vi "Interpret Driver Controls.vi"() -> ()   [LabVIEW 2018]
uses:
  <vilib>/Rock Robotics/WPI/DriverStation/WPI_DriverStationDerivedRobotMode.ctl
  Robot Global Data.vi
  SubSystems/Controllers/Driver Controller/Driver Controller Global.vi
  SubSystems/Drive Train/Drive Train Global.vi
  SubSystems/Lift/Lift Global.vi
  SubSystems/Controllers/Manipulator Controlller/Manipulator Controller Global.vi
  SubSystems/HAB Climber/HAB Climber Global.vi
  <vilib>/addons/control/pid/pid.llb/PID (DBL).vi
  SubSystems/Cargo Intake/Cargo Intake Global.vi
  SubSystems/Hatch Panel Intake/Hatch Panel Intake Global.vi
  <vilib>/addons/control/pid/NI_PID_pid.lvlib
panel:
  in  "Last Move Deadband":u32=500
  in  "Last Time Auto":u32=1171826
  in  "Camera Tracking":T1={"proportional gain (Kc)"=0.06, "integral time (Ti, min)"=0.0, "derivative time (Td, min)"=0.0}
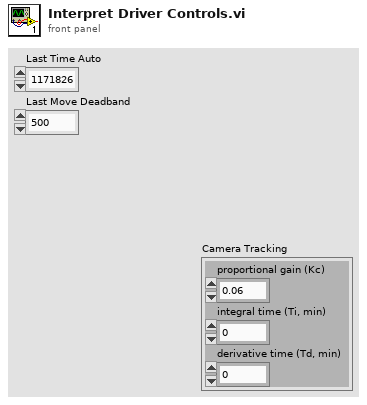
[diagram p1: front panel]
types:
  T1 = cluster{"proportional gain (Kc)":dbl, "integral time (Ti, min)":dbl, "derivative time (Td, min)":dbl}
  T2 = enum16{"Manual", "Hatch Panel Zone 1", "Hatch Panel Zone 2", "Hatch Panel Zone 3", "Cargo Zone 1", "Cargo Zone 2", "Cargo Zone 3", "Cargo Ship Zone"}
  T3 = enum16{"Hatch Panel Zone 1", "Hatch Panel Zone 2", "Hatch Panel Zone 3", "Cargo Zone 1", "Cargo Zone 2", "Cargo Zone 3", "Cargo Ship Zone"}
  T4 = cluster{"Rollover":dbl, "Yaw":dbl, "Cont Yaw":dbl}
  T5 = typedef "WPI_DriverStationDerivedRobotMode.ctl" = enum16{"Init", "Execute", "Stop"}
  T6 = cluster{"offsetAngle H":dbl, "offsetAngle V":dbl, "area":dbl, "skew":dbl, "validTarget":dbl, "latency":dbl}
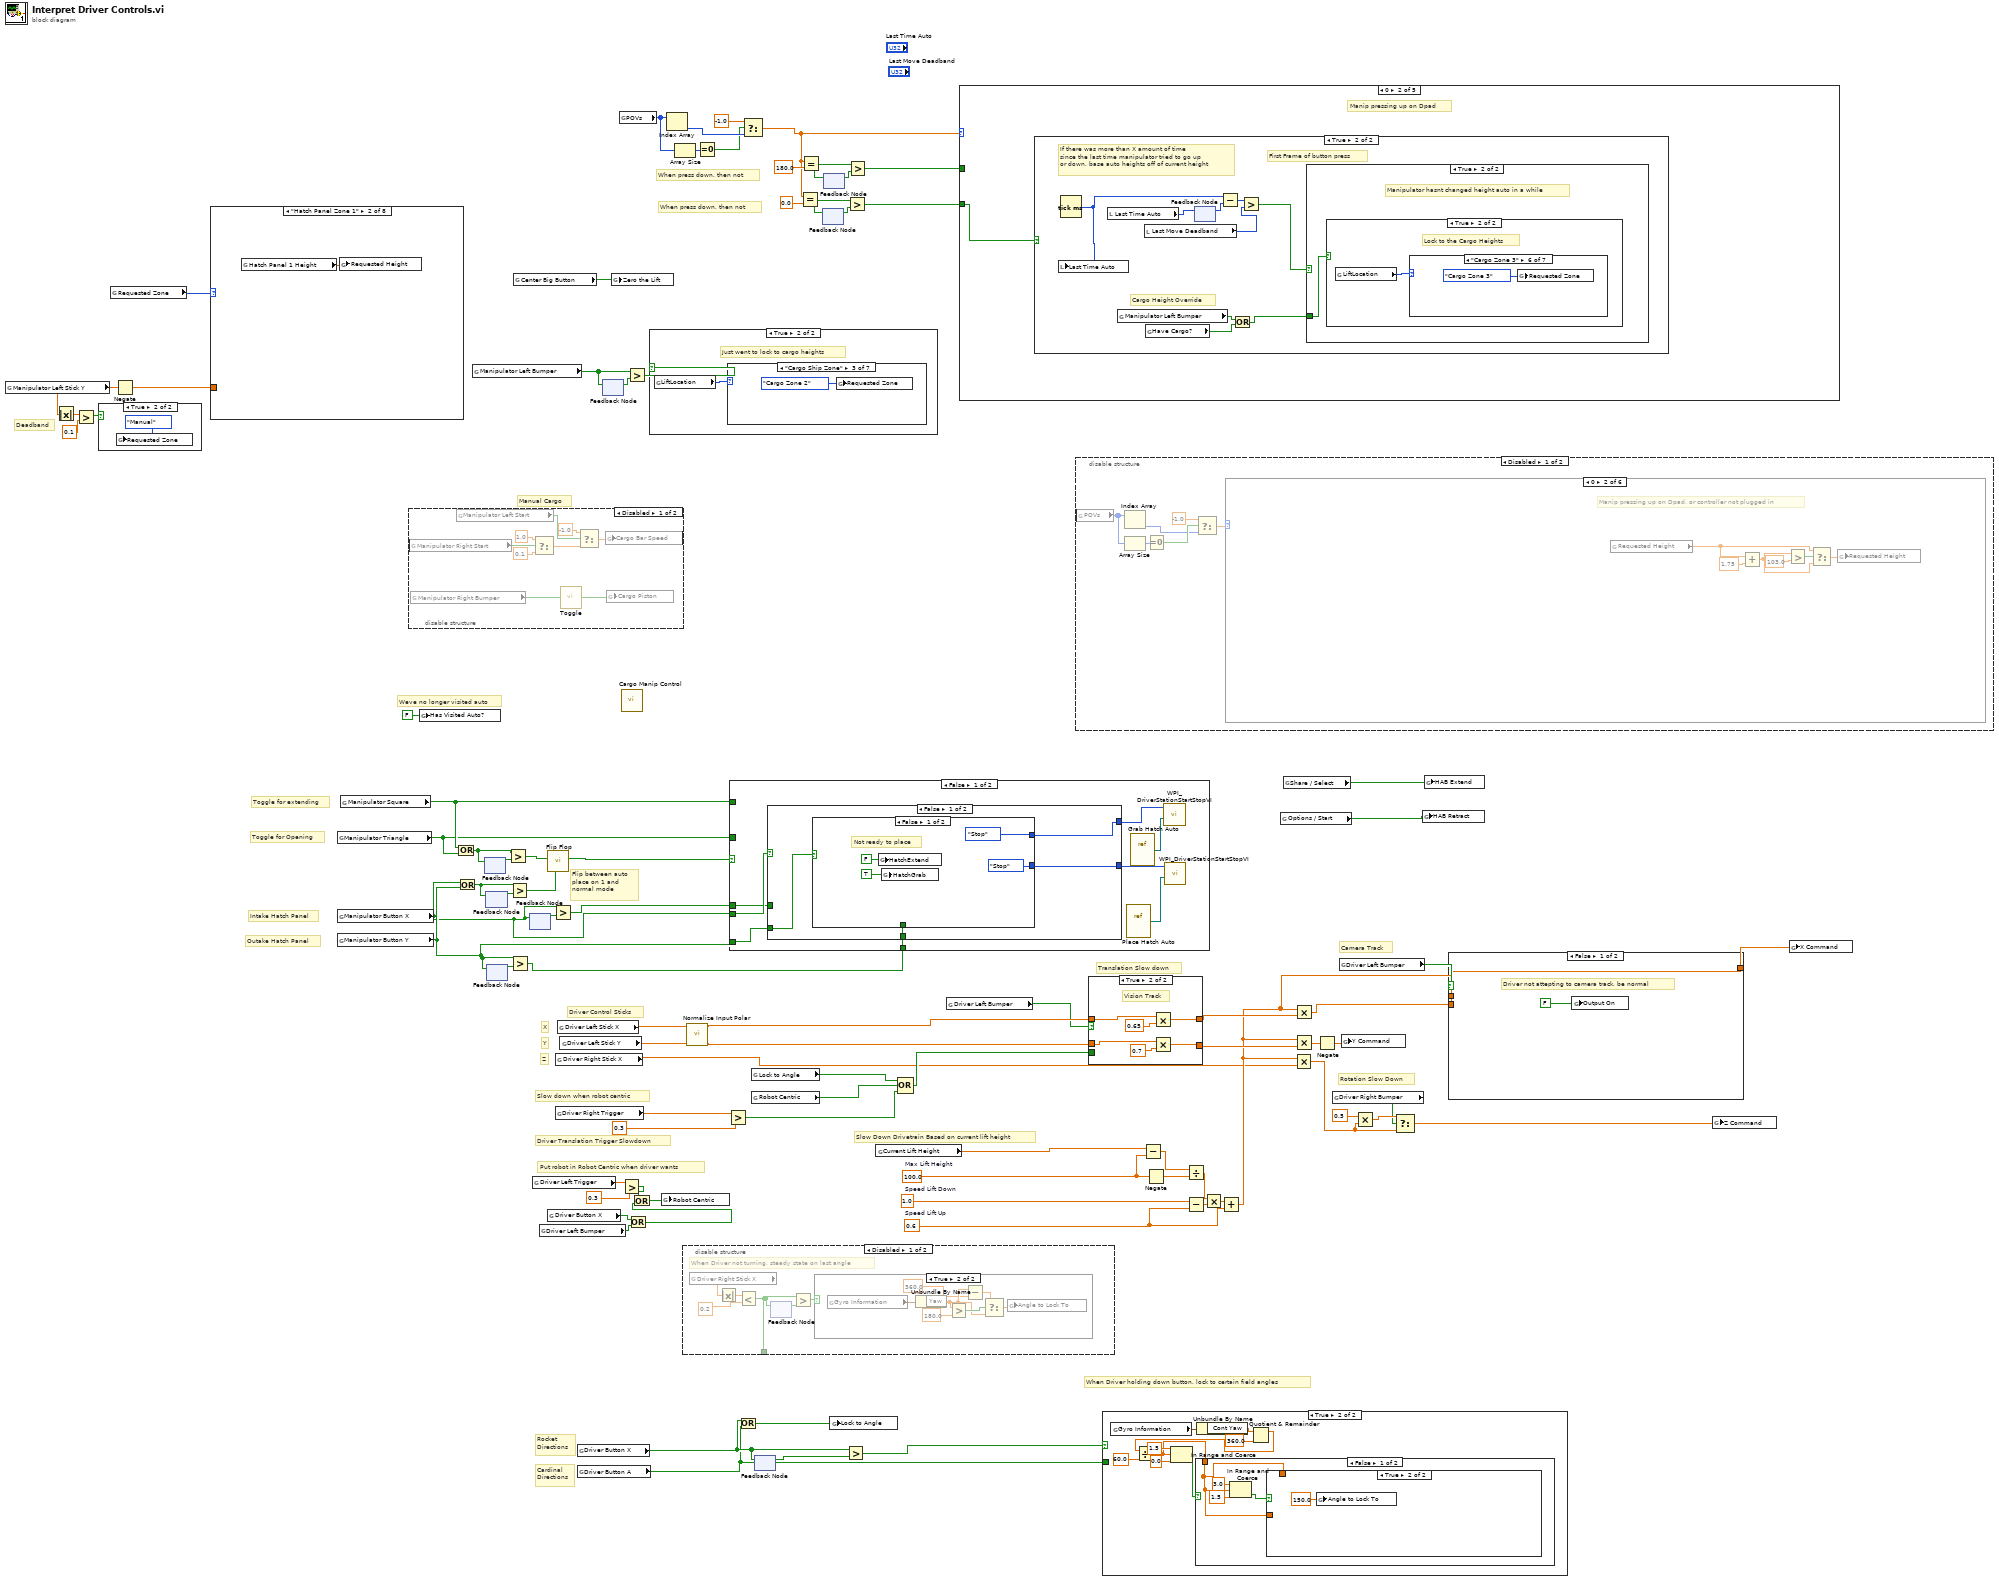
[diagram p0: block diagram]
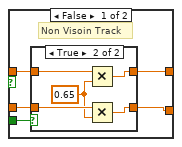
[diagram p2: hidden frame]
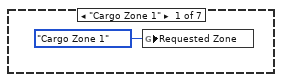
[diagram p5: hidden frame]
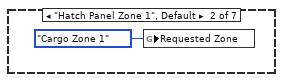
[diagram p6: hidden frame]
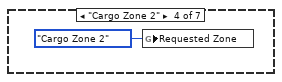
[diagram p7: hidden frame]
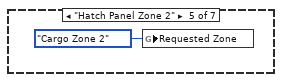
[diagram p8: hidden frame]
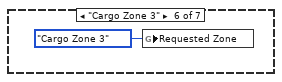
[diagram p9: hidden frame]
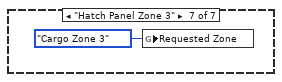
[diagram p10: hidden frame]
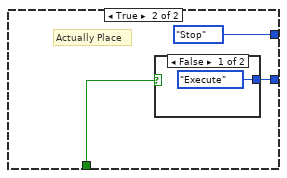
[diagram p11: hidden frame]
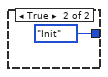
[diagram p12: hidden frame]
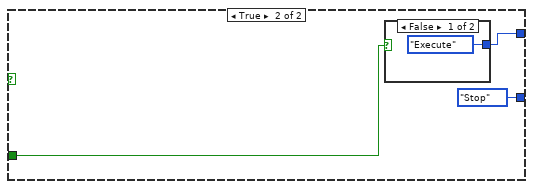
[diagram p13: hidden frame]
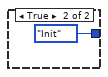
[diagram p14: hidden frame]
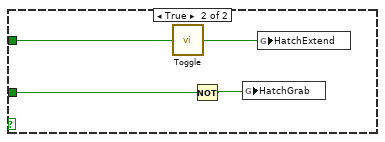
[diagram p15: hidden frame]
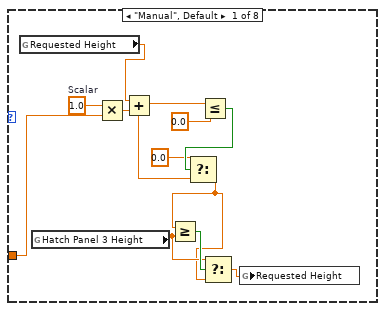
[diagram p17: hidden frame]
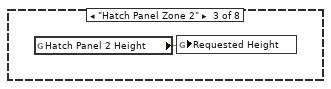
[diagram p18: hidden frame]
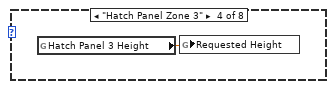
[diagram p19: hidden frame]
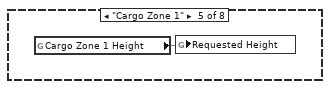
[diagram p20: hidden frame]
diagram:
  w69 = 0.6  # Speed Lift Up
  w73 = 1.0  # Speed Lift Down
  w67 = 100.0  # Max Lift Height
  # "Toggle for Opening"
  # "Toggle for extending"
  # "Outake Hatch Panel"
  # "Intake Hatch Panel"
  # "Flip between auto\nplace on 1 and \nnormal mode"
  # "When press down, then not"
  # "When press down, then not"
  # "Deadband"
  # "Manual Cargo"
  # "Weve no longer visited auto"
  # "Camera Track"
  # "Rotation Slow Down"
  # "Rocket\nDirections"
  # "Cardinal\nDirections"
  # "When Driver holding down button, lock to certain field angles"
  # "Slow Down Drivetrain Based on current lift height"
  # "Put robot in Robot Centric when driver wants"
  # "Slow down when robot centric"
  # "Driver Translation Trigger Slowdown"
  # "Translation Slow down"
  # "Z"
  # "Y"
  # "X"
  # "Driver Control Sticks"
  n1 = global read "Manipulator Controller Global.vi" "Manipulator Left Stick Y"() -> (w38:dbl)
  n2 = Absolute Value(x=w38) -> (abs(x)=w41:dbl)
  n3 = Greater?(x=w41, y=0.1) -> (0:w39:bool)
  n4 = case shown="True" w39 {
    frame False {
    }
    frame True {
      n5 = global write "Lift Global.vi" "Requested Zone"(T2."Manual" ("Requested Zone")) -> ()
    }
  }
  n6 = global read "Lift Global.vi" "Requested Zone"() -> (w42:T2)
  n7 = Negate(x=w38) -> (-x=w37:dbl)
  n8 = case shown="\"Hatch Panel Zone 1\"" w42 {
    tunnel: w37 -> [w99 _ _ _ _ _ _ _]
    frame "Manual", Default {
      w98 = 1.0  # Scalar
      n9 = global read "Lift Global.vi" "Requested Height"() -> (w101:dbl)
      n10 = global read "Lift Global.vi" "Hatch Panel 3 Height"() -> (w92:dbl)
      n11 = Multiply(x=w98, y=w99) -> (x*y=w100:dbl)
      n12 = Add(x=w101, y=w100) -> (x+y=w94:dbl)
      n13 = Less Or Equal?(x=w94, y=0.0) -> (x <= y?=w96:bool)
      n14 = Select(t=0.0, s=w96, f=w94) -> (s? t:f=w91:dbl)
      n15 = Greater Or Equal?(x=w91, y=w92) -> (x >= y?=w93:bool)
      n16 = Select(t=w92, s=w93, f=w91) -> (s? t:f=w90:dbl)
      n17 = global write "Lift Global.vi" "Requested Height"(w90) -> ()
    }
    frame "Hatch Panel Zone 1" {
      n18 = global read "Lift Global.vi" "Hatch Panel 1 Height"() -> (w102:dbl)
      n19 = global write "Lift Global.vi" "Requested Height"(w102) -> ()
    }
    frame "Hatch Panel Zone 2" {
      n20 = global read "Lift Global.vi" "Hatch Panel 2 Height"() -> (w103:dbl)
      n21 = global write "Lift Global.vi" "Requested Height"(w103) -> ()
    }
    frame "Hatch Panel Zone 3" {
      n22 = global read "Lift Global.vi" "Hatch Panel 3 Height"() -> (w104:dbl)
      n23 = global write "Lift Global.vi" "Requested Height"(w104) -> ()
    }
    frame "Cargo Zone 1" {
      n24 = global read "Lift Global.vi" "Cargo Zone 1 Height"() -> (w105:dbl)
      n25 = global write "Lift Global.vi" "Requested Height"(w105) -> ()
    }
    frame "Cargo Zone 2" {
      n26 = global read "Lift Global.vi" "Cargo Zone 2 Height"() -> (w106:dbl)
      n27 = global write "Lift Global.vi" "Requested Height"(w106) -> ()
    }
    frame "Cargo Zone 3" {
      n28 = global read "Lift Global.vi" "Cargo Zone 3 Height"() -> (w107:dbl)
      n29 = global write "Lift Global.vi" "Requested Height"(w107) -> ()
    }
    frame "Cargo Ship Zone" {
      n30 = global read "Lift Global.vi" "Cargo Ship Height"() -> (w108:dbl)
      n31 = global write "Lift Global.vi" "Requested Height"(w108) -> ()
    }
  }
  n32 = global read "Manipulator Controller Global.vi" "Manipulator Triangle"() -> (w24:bool)
  n33 = global read "Manipulator Controller Global.vi" "Manipulator Button X"() -> (w11:bool)
  n34 = global read "Manipulator Controller Global.vi" "Manipulator Button Y"() -> (w14:bool)
  n35 = global read "Manipulator Controller Global.vi" "Manipulator Square"() -> (w25:bool)
  n36 = disable-structure shown="Disabled" {
    frame Disabled {
      n37 = global read "Manipulator Controller Global.vi" "Manipulator Right Start"() -> (w114:bool)
      n38 = global read "Manipulator Controller Global.vi" "Manipulator Right Bumper"() -> (w117:bool)
      n39 = global read "Manipulator Controller Global.vi" "Manipulator Left Start"() -> (w113:bool)
      n40 = Select(t=1.0, s=w114, f=0.1) -> (s? t:f=w112:dbl)
      n41 = call "Toggle.vi"("Input"=w117) -> ("Output"=w116:bool)
      n42 = Select(t=-1.0, s=w113, f=w112) -> (s? t:f=w115:dbl)
      n43 = global write "Cargo Intake Global.vi" "Cargo Bar Speed"(w115) -> ()
      n44 = global write "Cargo Intake Global.vi" "Cargo Piston"(w116) -> ()
    }
    frame Enabled {
    }
  }
  n45 = global write "Robot Global Data.vi" "Has Visited Auto?"(FALSE ("Has Visited Auto?")) -> ()
  n46 = Or(x=w25, y=w24) -> (x .or. y?=w22:bool)
  n47 = Or(x=w11, y=w14) -> (x .or. y?=w19:bool)
  n48 = global read "Manipulator Controller Global.vi" "Manipulator Left Bumper"() -> (w8:bool)
  n49 = feedback-in #1(w22) -> ()
  n50 = feedback #1() -> (w23:bool)  [unwired: 1 in]
  n51 = feedback #2() -> (w20:bool)  [unwired: 1 in]
  n52 = feedback-in #2(w19) -> ()
  n53 = feedback #3() -> (w16:bool)  [unwired: 1 in]
  n54 = feedback-in #3(w14) -> ()
  n55 = Greater?(x=w22, y=w23) -> (0:w21:bool)
  n56 = Greater?(x=w19, y=w20) -> (0:w18:bool)
  n57 = Greater?(x=w14, y=w16) -> (0:w15:bool)
  n58 = global read "Manipulator Controller Global.vi" "Center Big Button"() -> (w2:bool)
  n59 = feedback #4() -> (w12:bool)  [unwired: 1 in]
  n60 = feedback-in #4(w11) -> ()
  n61 = global read "Driver Controller Global.vi" "Driver Left Trigger"() -> (w85:dbl)
  n62 = global read "Driver Controller Global.vi" "Driver Left Bumper"() -> (w52:bool)
  n63 = call "Flip Flop.vi"("Line 2"=w18, "Line 1"=w21) -> ("Switch"=w17:bool)  [unwired: 9 in]
  n64 = global read "Driver Controller Global.vi" "Driver Button X"() -> (w53:bool)
  n65 = Greater?(x=w11, y=w12) -> (0:w10:bool)
  n66 = global read "Driver Controller Global.vi" "Driver Right Trigger"() -> (w88:dbl)
  n67 = global read "Driver Controller Global.vi" "Driver Right Stick X"() -> (w13:dbl)
  n68 = global read "Driver Controller Global.vi" "Driver Left Stick X"() -> (w4:dbl)
  n69 = global read "Driver Controller Global.vi" "Driver Left Stick Y"() -> (w3:dbl)
  n70 = global read "Driver Controller Global.vi" "Driver Button X"() -> (w65:bool)
  n71 = global read "Driver Controller Global.vi" "Driver Button A"() -> (w63:bool)
  n72 = feedback #5() -> (w9:bool)  [unwired: 1 in]
  n73 = feedback-in #5(w8) -> ()
  n74 = global write "Lift Global.vi" "Zero the Lift"(w2) -> ()
  n75 = global read "Manipulator Controller Global.vi" "POVs"() -> (w46:i16[])
  n76 = call "Cargo Manip Control.vi"() -> ()  [unwired: 12 in]
  n77 = Greater?(x=w85, y=0.3) -> (0:w61:bool)
  n78 = Greater?(x=w8, y=w9) -> (0:w7:bool)
  n79 = Or(x=w53, y=w52) -> (x .or. y?=w54:bool)
  n80 = Or(x=w61, y=w54) -> (x .or. y?=w59:bool)
  n81 = case shown="True" w7 {
    frame False {
    }
    frame True {
      # "Just went to lock to cargo heights"
      n82 = global read "Lift Global.vi" "LiftLocation"() -> (w118:T3)
      n83 = case shown="\"Cargo Ship Zone\"" w118 {
        frame "Cargo Zone 1" {
          n84 = global write "Lift Global.vi" "Requested Zone"(T2."Cargo Zone 1" ("Requested Zone")) -> ()
        }
        frame "Hatch Panel Zone 1", Default {
          n85 = global write "Lift Global.vi" "Requested Zone"(T2."Cargo Zone 1" ("Requested Zone")) -> ()
        }
        frame "Cargo Ship Zone" {
          n86 = global write "Lift Global.vi" "Requested Zone"(T2."Cargo Zone 2" ("Requested Zone")) -> ()
        }
        frame "Cargo Zone 2" {
          n87 = global write "Lift Global.vi" "Requested Zone"(T2."Cargo Zone 2" ("Requested Zone")) -> ()
        }
        frame "Hatch Panel Zone 2" {
          n88 = global write "Lift Global.vi" "Requested Zone"(T2."Cargo Zone 2" ("Requested Zone")) -> ()
        }
        frame "Cargo Zone 3" {
          n89 = global write "Lift Global.vi" "Requested Zone"(T2."Cargo Zone 3" ("Requested Zone")) -> ()
        }
        frame "Hatch Panel Zone 3" {
          n90 = global write "Lift Global.vi" "Requested Zone"(T2."Cargo Zone 3" ("Requested Zone")) -> ()
        }
      }
    }
  }
  n91 = global write "Drive Train Global.vi" "Robot Centric"(w59) -> ()
  n92 = Index Array(array=w46) -> (element=w43:i16)  [unwired: 1 in]
  n93 = Array Size(array=w46) -> (size(s)=w45:i32)
  n94 = disable-structure shown="Disabled" {
    disable-tunnel: [w126 _] -> _
    frame Disabled {
      # "When Driver not turning, steady state on last angle"
      n95 = global read "Driver Controller Global.vi" "Driver Right Stick X"() -> (w127:dbl)
      n96 = Absolute Value(x=w127) -> (abs(x)=w131:dbl)
      n97 = Less?(x=w131, y=0.2) -> (x < y?=w126:bool)
      n98 = feedback #6() -> (w129:bool)  [unwired: 1 in]
      n99 = feedback-in #6(w126) -> ()
      n100 = Greater?(x=w126, y=w129) -> (0:w128:bool)
      n101 = case shown="True" w128 {
        frame False {
        }
        frame True {
          n102 = global read "Drive Train Global.vi" "Gyro Information"() -> (w138:T4)
          n103 = Unbundle By Name(w138) -> ("Yaw"=w135:dbl)
          n104 = Greater?(x=w135, y=180.0) -> (0:w136:bool)
          n105 = Subtract(x=w135, y=360.0) -> (x-y=w133:dbl)
          n106 = Select(t=w133, s=w136, f=w135) -> (s? t:f=w132:dbl)
          n107 = global write "Drive Train Global.vi" "Angle to Lock To"(w132) -> ()
        }
      }
    }
    frame Enabled {
    }
  }
  n108 = call "Normalize Input Polar.vi"("V Input"=w3, "U Input"=w4) -> ("Y Output"=w5:dbl, "X Output"=w6:dbl)  [unwired: 8 in]
  n109 = Equal To 0?(x=w45) -> (x = 0?=w36:bool)
  n110 = Greater?(x=w88, y=0.3) -> (0:w80:bool)
  n111 = case shown="False" w17 {
    tunnel: w24 -> [_ w166]
    tunnel: w25 -> [_ w167]
    tunnel: w11 -> [w146 _]
    tunnel: w15 -> [w143 _]
    tunnel: w14 -> [w142 _]
    tunnel: w10 -> [w139 _]
    frame False {
      n112 = case shown="False" w146 {
        tunnel: [w150 WPI_DriverStationDerivedRobotMode."Stop" ("Call Context")] -> w144
        tunnel: w143 -> [w149 _]
        tunnel: w142 -> [w148 _]
        tunnel: [w147 w161] -> w140
        tunnel: w139 -> [_ w160]
        frame False {
          n113 = case shown="False" w148 {
            tunnel: [WPI_DriverStationDerivedRobotMode."Stop" ("Call Context") w157] -> w150
            tunnel: w149 -> [_ w156]
            tunnel: [WPI_DriverStationDerivedRobotMode."Stop" ("Call Context") WPI_DriverStationDerivedRobotMode."Stop" ("Call Context")] -> w147
            frame False {
              # "Not ready to place"
              n114 = global write "Hatch Panel Intake Global.vi" "HatchExtend"(FALSE ("HatchExtend")) -> ()
              n115 = global write "Hatch Panel Intake Global.vi" "HatchGrab"(TRUE ("HatchExtend")) -> ()
            }
            frame True {
              # "Actually Place"
              n116 = case shown="False" w156 {
                tunnel: [WPI_DriverStationDerivedRobotMode."Execute" ("Call Context") WPI_DriverStationDerivedRobotMode."Init" ("Call Context")] -> w157
                frame False {
                }
                frame True {
                }
              }
            }
          }
        }
        frame True {
          n117 = case shown="False" w160 {
            tunnel: [WPI_DriverStationDerivedRobotMode."Execute" ("Call Context") WPI_DriverStationDerivedRobotMode."Init" ("Call Context")] -> w161
            frame False {
            }
            frame True {
            }
          }
        }
      }
      n118 = vi-ref "Place Hatch Auto.vi"() -> (w145:refnum<vi>)
      n119 = vi-ref "Grab Hatch Auto.vi"() -> (w141:refnum<vi>)
      n120 = call <vilib>:"WPI_DriverStationStartStopVI.vi"("VI in"=w141, "Call Context"=w140) -> ()  [unwired: 10 in]
      n121 = call <vilib>:"WPI_DriverStationStartStopVI.vi"("VI in"=w145, "Call Context"=w144) -> ()  [unwired: 10 in]
    }
    frame True {
      n122 = call "Toggle.vi"("Input"=w167) -> ("Output"=w168:bool)
      n123 = Not(x=w166) -> (.not. x?=w165:bool)
      n124 = global write "Hatch Panel Intake Global.vi" "HatchGrab"(w165) -> ()
      n125 = global write "Hatch Panel Intake Global.vi" "HatchExtend"(w168) -> ()
    }
  }
  n126 = Or(x=w65, y=w63) -> (x .or. y?=w62:bool)
  n127 = Select(t=-1.0, s=w36, f=w43) -> (s? t:f=w28:dbl)
  n128 = global read "Drive Train Global.vi" "Lock to Angle"() -> (w60:bool)
  n129 = global read "Drive Train Global.vi" "Robot Centric"() -> (w79:bool)
  n130 = feedback #7() -> (w66:bool)  [unwired: 1 in]
  n131 = feedback-in #7(w65) -> ()
  n132 = Equal?(x=w28, y=0.0) -> (x = y?=w31:bool)
  n133 = Equal?(x=w28, y=180.0) -> (x = y?=w33:bool)
  n134 = feedback #8() -> (w30:bool)  [unwired: 1 in]
  n135 = feedback-in #8(w31) -> ()
  n136 = feedback-in #9(w33) -> ()
  n137 = feedback #9() -> (w34:bool)  [unwired: 1 in]
  n138 = global write "Drive Train Global.vi" "Lock to Angle"(w62) -> ()
  n139 = Greater?(x=w65, y=w66) -> (0:w64:bool)
  n140 = Greater?(x=w31, y=w30) -> (0:w27:bool)
  n141 = Greater?(x=w33, y=w34) -> (0:w32:bool)
  n142 = global read "Lift Global.vi" "Current Lift Height"() -> (w75:dbl)
  n143 = Compound Arithmetic op=OR(w60, w79, w80) -> (w78:bool)
  n144 = global read "Driver Controller Global.vi" "Driver Left Bumper"() -> (w1:bool)
  n145 = case shown="0" w28 {
    tunnel: w32 -> [_ _ w213 _ _]
    tunnel: w27 -> [_ w169 _ _ _]
    frame -1, Default {
      # "Nothing on the D-Pad is pressed!"
    }
    frame 0 {
      # "Manip pressing up on Dpad"
      n146 = case shown="True" w169 {
        frame False {
          # "Still pressing button, do nothing"
        }
        frame True {
          # "Cargo Height Override"
          # "First Frame of button press"
          # "If there was more than X amount of time\nsince the last time manipulator tried to go up\nor down, base auto heights off of current height"
          n147 = Tick Count (ms)() -> (millisecond timer value=w175:u32)
          n148 = local write "Last Time Auto"(w175) -> ()
          n149 = local read "Last Time Auto"() -> (w174:u32)
          n150 = global read "Manipulator Controller Global.vi" "Manipulator Left Bumper"() -> (w172:bool)
          n151 = local read "Last Move Deadband"() -> (w176:u32)
          n152 = global read "Cargo Intake Global.vi" "Have Cargo?"() -> (w170:bool)
          n153 = feedback #10() -> (w173:u32)  [unwired: 1 in]
          n154 = feedback-in #10(w174) -> ()
          n155 = Subtract(x=w175, y=w173) -> (x-y=w178:u32)
          n156 = Or(x=w172, y=w170) -> (x .or. y?=w171:bool)
          n157 = Greater?(x=w178, y=w176) -> (0:w177:bool)
          n158 = case shown="True" w177 {
            tunnel: w171 -> [w179 w196]
            frame False {
              # "Manipulator is still changing height to go to"
              n159 = case shown="False" w179 {
                frame False {
                  # "Lock to the Hatch Heights"
                  n160 = global read "Lift Global.vi" "Requested Zone"() -> (w180:T2)
                  n161 = case shown="\"Hatch Panel Zone 3\"" w180 {
                    frame "Manual" {
                    }
                    frame "Cargo Zone 1" {
                      n162 = global write "Lift Global.vi" "Requested Zone"(T2."Hatch Panel Zone 1" ("Requested Zone")) -> ()
                    }
                    frame "Hatch Panel Zone 1", Default {
                      n163 = global write "Lift Global.vi" "Requested Zone"(T2."Hatch Panel Zone 2" ("Requested Zone")) -> ()
                    }
                    frame "Cargo Ship Zone" {
                      n164 = global write "Lift Global.vi" "Requested Zone"(T2."Hatch Panel Zone 2" ("Requested Zone")) -> ()
                    }
                    frame "Cargo Zone 2" {
                      n165 = global write "Lift Global.vi" "Requested Zone"(T2."Hatch Panel Zone 2" ("Requested Zone")) -> ()
                    }
                    frame "Hatch Panel Zone 2" {
                      n166 = global write "Lift Global.vi" "Requested Zone"(T2."Hatch Panel Zone 3" ("Requested Zone")) -> ()
                    }
                    frame "Cargo Zone 3" {
                      n167 = global write "Lift Global.vi" "Requested Zone"(T2."Hatch Panel Zone 3" ("Requested Zone")) -> ()
                    }
                    frame "Hatch Panel Zone 3" {
                      n168 = global write "Lift Global.vi" "Requested Zone"(T2."Hatch Panel Zone 3" ("Requested Zone")) -> ()
                    }
                  }
                }
                frame True {
                  # "Lock to the Cargo Heights"
                  n169 = global read "Lift Global.vi" "Requested Zone"() -> (w188:T2)
                  n170 = case shown="\"Manual\"" w188 {
                    frame "Manual" {
                    }
                    frame "Cargo Zone 1" {
                      n171 = global write "Lift Global.vi" "Requested Zone"(T2."Cargo Zone 2" ("Requested Zone")) -> ()
                    }
                    frame "Hatch Panel Zone 1", Default {
                      n172 = global write "Lift Global.vi" "Requested Zone"(T2."Cargo Zone 2" ("Requested Zone")) -> ()
                    }
                    frame "Cargo Ship Zone" {
                      n173 = global write "Lift Global.vi" "Requested Zone"(T2."Cargo Zone 2" ("Requested Zone")) -> ()
                    }
                    frame "Cargo Zone 2" {
                      n174 = global write "Lift Global.vi" "Requested Zone"(T2."Cargo Zone 3" ("Requested Zone")) -> ()
                    }
                    frame "Hatch Panel Zone 2" {
                      n175 = global write "Lift Global.vi" "Requested Zone"(T2."Cargo Zone 3" ("Requested Zone")) -> ()
                    }
                    frame "Cargo Zone 3" {
                      n176 = global write "Lift Global.vi" "Requested Zone"(T2."Cargo Zone 3" ("Requested Zone")) -> ()
                    }
                    frame "Hatch Panel Zone 3" {
                      n177 = global write "Lift Global.vi" "Requested Zone"(T2."Cargo Zone 3" ("Requested Zone")) -> ()
                    }
                  }
                }
              }
            }
            frame True {
              # "Manipulator hasnt changed height auto in a while"
              n178 = case shown="True" w196 {
                frame False {
                  # "Lock to the Hatch Heights"
                  n179 = global read "Lift Global.vi" "LiftLocation"() -> (w197:T3)
                  n180 = case shown="\"Cargo Zone 1\"" w197 {
                    frame "Cargo Zone 1" {
                      n181 = global write "Lift Global.vi" "Requested Zone"(T2."Hatch Panel Zone 1" ("Requested Zone")) -> ()
                    }
                    frame "Hatch Panel Zone 1", Default {
                      n182 = global write "Lift Global.vi" "Requested Zone"(T2."Hatch Panel Zone 2" ("Requested Zone")) -> ()
                    }
                    frame "Cargo Ship Zone" {
                      n183 = global write "Lift Global.vi" "Requested Zone"(T2."Hatch Panel Zone 2" ("Requested Zone")) -> ()
                    }
                    frame "Cargo Zone 2" {
                      n184 = global write "Lift Global.vi" "Requested Zone"(T2."Hatch Panel Zone 2" ("Requested Zone")) -> ()
                    }
                    frame "Hatch Panel Zone 2" {
                      n185 = global write "Lift Global.vi" "Requested Zone"(T2."Hatch Panel Zone 3" ("Requested Zone")) -> ()
                    }
                    frame "Cargo Zone 3" {
                      n186 = global write "Lift Global.vi" "Requested Zone"(T2."Hatch Panel Zone 3" ("Requested Zone")) -> ()
                    }
                    frame "Hatch Panel Zone 3" {
                      n187 = global write "Lift Global.vi" "Requested Zone"(T2."Hatch Panel Zone 3" ("Requested Zone")) -> ()
                    }
                  }
                }
                frame True {
                  # "Lock to the Cargo Heights"
                  n188 = global read "Lift Global.vi" "LiftLocation"() -> (w205:T3)
                  n189 = case shown="\"Cargo Zone 3\"" w205 {
                    frame "Cargo Zone 1" {
                      n190 = global write "Lift Global.vi" "Requested Zone"(T2."Cargo Zone 2" ("Requested Zone")) -> ()
                    }
                    frame "Hatch Panel Zone 1", Default {
                      n191 = global write "Lift Global.vi" "Requested Zone"(T2."Cargo Zone 2" ("Requested Zone")) -> ()
                    }
                    frame "Cargo Ship Zone" {
                      n192 = global write "Lift Global.vi" "Requested Zone"(T2."Cargo Zone 2" ("Requested Zone")) -> ()
                    }
                    frame "Cargo Zone 2" {
                      n193 = global write "Lift Global.vi" "Requested Zone"(T2."Cargo Zone 3" ("Requested Zone")) -> ()
                    }
                    frame "Hatch Panel Zone 2" {
                      n194 = global write "Lift Global.vi" "Requested Zone"(T2."Cargo Zone 3" ("Requested Zone")) -> ()
                    }
                    frame "Cargo Zone 3" {
                      n195 = global write "Lift Global.vi" "Requested Zone"(T2."Cargo Zone 3" ("Requested Zone")) -> ()
                    }
                    frame "Hatch Panel Zone 3" {
                      n196 = global write "Lift Global.vi" "Requested Zone"(T2."Cargo Zone 3" ("Requested Zone")) -> ()
                    }
                  }
                }
              }
            }
          }
        }
      }
    }
    frame 180 {
      # "Manip pressing down on Dpad"
      n197 = case shown="True" w213 {
        frame False {
          # "Still pressing button, do nothing"
        }
        frame True {
          # "Cargo Height Override"
          # "First frame of button press"
          # "If there was more than X amount of time\nsince the last time manipulator tried to go up\nor down, base auto heights off of current height"
          n198 = Tick Count (ms)() -> (millisecond timer value=w221:u32)
          n199 = local write "Last Time Auto"(w221) -> ()
          n200 = local read "Last Time Auto"() -> (w219:u32)
          n201 = global read "Manipulator Controller Global.vi" "Manipulator Left Bumper"() -> (w216:bool)
          n202 = local read "Last Move Deadband"() -> (w220:u32)
          n203 = global read "Cargo Intake Global.vi" "Have Cargo?"() -> (w215:bool)
          n204 = feedback #11() -> (w218:u32)  [unwired: 1 in]
          n205 = feedback-in #11(w219) -> ()
          n206 = Subtract(x=w221, y=w218) -> (x-y=w222:u32)
          n207 = Greater?(x=w222, y=w220) -> (0:w217:bool)
          n208 = Or(x=w216, y=w215) -> (x .or. y?=w214:bool)
          n209 = case shown="False" w217 {
            tunnel: w214 -> [w223 w240]
            frame False {
              # "Manipulator is still changing height to go to"
              n210 = case shown="False" w223 {
                frame False {
                  # "Lock to the Hatch Heights"
                  n211 = global read "Lift Global.vi" "Requested Zone"() -> (w224:T2)
                  n212 = case shown="\"Hatch Panel Zone 3\"" w224 {
                    frame "Manual" {
                    }
                    frame "Cargo Zone 1" {
                      n213 = global write "Lift Global.vi" "Requested Zone"(T2."Hatch Panel Zone 1" ("Requested Zone")) -> ()
                    }
                    frame "Hatch Panel Zone 1", Default {
                      n214 = global write "Lift Global.vi" "Requested Zone"(T2."Hatch Panel Zone 1" ("Requested Zone")) -> ()
                    }
                    frame "Cargo Ship Zone" {
                      n215 = global write "Lift Global.vi" "Requested Zone"(T2."Hatch Panel Zone 1" ("Requested Zone")) -> ()
                    }
                    frame "Cargo Zone 2" {
                      n216 = global write "Lift Global.vi" "Requested Zone"(T2."Hatch Panel Zone 1" ("Requested Zone")) -> ()
                    }
                    frame "Hatch Panel Zone 2" {
                      n217 = global write "Lift Global.vi" "Requested Zone"(T2."Hatch Panel Zone 1" ("Requested Zone")) -> ()
                    }
                    frame "Cargo Zone 3" {
                      n218 = global write "Lift Global.vi" "Requested Zone"(T2."Hatch Panel Zone 2" ("Requested Zone")) -> ()
                    }
                    frame "Hatch Panel Zone 3" {
                      n219 = global write "Lift Global.vi" "Requested Zone"(T2."Hatch Panel Zone 2" ("Requested Zone")) -> ()
                    }
                  }
                }
                frame True {
                  # "Lock to the Cargo Heights"
                  n220 = global read "Lift Global.vi" "Requested Zone"() -> (w232:T2)
                  n221 = case shown="\"Manual\"" w232 {
                    frame "Manual" {
                    }
                    frame "Cargo Zone 1" {
                      n222 = global write "Lift Global.vi" "Requested Zone"(T2."Cargo Zone 1" ("Requested Zone")) -> ()
                    }
                    frame "Hatch Panel Zone 1", Default {
                      n223 = global write "Lift Global.vi" "Requested Zone"(T2."Cargo Zone 1" ("Requested Zone")) -> ()
                    }
                    frame "Cargo Ship Zone" {
                      n224 = global write "Lift Global.vi" "Requested Zone"(T2."Cargo Zone 1" ("Requested Zone")) -> ()
                    }
                    frame "Cargo Zone 2" {
                      n225 = global write "Lift Global.vi" "Requested Zone"(T2."Cargo Zone 1" ("Requested Zone")) -> ()
                    }
                    frame "Hatch Panel Zone 2" {
                      n226 = global write "Lift Global.vi" "Requested Zone"(T2."Cargo Zone 2" ("Requested Zone")) -> ()
                    }
                    frame "Cargo Zone 3" {
                      n227 = global write "Lift Global.vi" "Requested Zone"(T2."Cargo Zone 2" ("Requested Zone")) -> ()
                    }
                    frame "Hatch Panel Zone 3" {
                      n228 = global write "Lift Global.vi" "Requested Zone"(T2."Cargo Zone 3" ("Requested Zone")) -> ()
                    }
                  }
                }
              }
            }
            frame True {
              # "Manipulator hasnt changed height auto in a while"
              n229 = case shown="False" w240 {
                frame False {
                  # "Lock to the Hatch Heights"
                  n230 = global read "Lift Global.vi" "LiftLocation"() -> (w241:T3)
                  n231 = case shown="\"Hatch Panel Zone 3\"" w241 {
                    frame "Cargo Zone 1" {
                      n232 = global write "Lift Global.vi" "Requested Zone"(T2."Hatch Panel Zone 1" ("Requested Zone")) -> ()
                    }
                    frame "Hatch Panel Zone 1", Default {
                      n233 = global write "Lift Global.vi" "Requested Zone"(T2."Hatch Panel Zone 1" ("Requested Zone")) -> ()
                    }
                    frame "Cargo Ship Zone" {
                      n234 = global write "Lift Global.vi" "Requested Zone"(T2."Hatch Panel Zone 1" ("Requested Zone")) -> ()
                    }
                    frame "Cargo Zone 2" {
                      n235 = global write "Lift Global.vi" "Requested Zone"(T2."Hatch Panel Zone 1" ("Requested Zone")) -> ()
                    }
                    frame "Hatch Panel Zone 2" {
                      n236 = global write "Lift Global.vi" "Requested Zone"(T2."Hatch Panel Zone 1" ("Requested Zone")) -> ()
                    }
                    frame "Cargo Zone 3" {
                      n237 = global write "Lift Global.vi" "Requested Zone"(T2."Hatch Panel Zone 2" ("Requested Zone")) -> ()
                    }
                    frame "Hatch Panel Zone 3" {
                      n238 = global write "Lift Global.vi" "Requested Zone"(T2."Hatch Panel Zone 2" ("Requested Zone")) -> ()
                    }
                  }
                }
                frame True {
                  # "Lock to the Cargo Heights"
                  n239 = global read "Lift Global.vi" "LiftLocation"() -> (w249:T3)
                  n240 = case shown="\"Hatch Panel Zone 3\"" w249 {
                    frame "Cargo Zone 1" {
                      n241 = global write "Lift Global.vi" "Requested Zone"(T2."Cargo Zone 1" ("Requested Zone")) -> ()
                    }
                    frame "Hatch Panel Zone 1", Default {
                      n242 = global write "Lift Global.vi" "Requested Zone"(T2."Cargo Zone 1" ("Requested Zone")) -> ()
                    }
                    frame "Cargo Ship Zone" {
                      n243 = global write "Lift Global.vi" "Requested Zone"(T2."Cargo Zone 1" ("Requested Zone")) -> ()
                    }
                    frame "Cargo Zone 2" {
                      n244 = global write "Lift Global.vi" "Requested Zone"(T2."Cargo Zone 1" ("Requested Zone")) -> ()
                    }
                    frame "Hatch Panel Zone 2" {
                      n245 = global write "Lift Global.vi" "Requested Zone"(T2."Cargo Zone 2" ("Requested Zone")) -> ()
                    }
                    frame "Cargo Zone 3" {
                      n246 = global write "Lift Global.vi" "Requested Zone"(T2."Cargo Zone 2" ("Requested Zone")) -> ()
                    }
                    frame "Hatch Panel Zone 3" {
                      n247 = global write "Lift Global.vi" "Requested Zone"(T2."Cargo Zone 3" ("Requested Zone")) -> ()
                    }
                  }
                }
              }
            }
          }
        }
      }
    }
    frame 90 {
      # "Go to Cargo in Cargo Ship Height"
      # "Right on D-Pad"
      n248 = global write "Lift Global.vi" "Requested Zone"(T2."Cargo Ship Zone" ("Requested Zone")) -> ()
    }
    frame 270 {
      # "Go to Hatch Level 1 Height"
      # "Left on D-Pad"
      n249 = global write "Lift Global.vi" "Requested Zone"(T2."Hatch Panel Zone 1" ("Requested Zone")) -> ()
    }
  }
  n250 = disable-structure shown="Disabled" {
    frame Disabled {
      n251 = global read "Manipulator Controller Global.vi" "POVs"() -> (w264:i16[])
      n252 = Index Array(array=w264) -> (element=w259:i16)  [unwired: 1 in]
      n253 = Array Size(array=w264) -> (size(s)=w263:i32)
      n254 = Equal To 0?(x=w263) -> (x = 0?=w261:bool)
      n255 = Select(t=-1.0, s=w261, f=w259) -> (s? t:f=w262:dbl)
      n256 = case shown="0" w262 {
        frame -1 {
          # "If the value changed (manip pressed button)\nchange set lift height to match"
          # "When button goes from\nnot pressed to pressed"
          n257 = global read "Manipulator Controller Global.vi" "Manipulator Square"() -> (w270:bool)
          n258 = feedback #12() -> (w271:bool)  [unwired: 1 in]
          n259 = feedback-in #12(w270) -> ()
          n260 = Greater?(x=w270, y=w271) -> (0:w267:bool)
          n261 = feedback #13() -> (w265:dbl)  [unwired: 1 in]
          n262 = feedback #14() -> (w269:dbl)  [unwired: 1 in]
          n263 = case shown="False" w267 {
            tunnel: [w281 w296] -> w266
            tunnel: w269 -> [w282 w295]
            frame False {
              # "When button goes from\nnot pressed to pressed"
              n264 = global read "Manipulator Controller Global.vi" "Manipulator Triangle"() -> (w284:bool)
              n265 = feedback #15() -> (w283:bool)  [unwired: 1 in]
              n266 = feedback-in #15(w284) -> ()
              n267 = Greater?(x=w284, y=w283) -> (0:w280:bool)
              n268 = case shown="True" w280 {
                tunnel: w282 -> [w285 w287]
                tunnel: [w285 w289] -> w281
                frame False {
                }
                frame True {
                  # "If counter smaller than 5\nadd 1"
                  n269 = Less?(x=w287, y=5.0) -> (x < y?=w286:bool)
                  n270 = case shown="True" w286 {
                    tunnel: [w290 w292] -> w289
                    tunnel: w287 -> [w290 w291]
                    frame False {
                    }
                    frame True {
                      n271 = Increment(x=w291) -> (x+1=w292:dbl)
                    }
                  }
                }
              }
            }
            frame True {
              # "If counter bigger than 0\nsubtract 1"
              n272 = Greater?(x=w295, y=0.0) -> (0:w294:bool)
              n273 = case shown="False" w294 {
                tunnel: [0.0 ("y") w299] -> w296
                tunnel: w295 -> [_ w298]
                frame False {
                }
                frame True {
                  n274 = Decrement(x=w298) -> (x-1=w299:dbl)
                }
              }
            }
          }
          n275 = feedback-in #13(w266) -> ()
          n276 = Not Equal?(x=w266, y=w265) -> (x != y?=w268:bool)
          n277 = case shown="True" w268 {
            tunnel: w266 -> [_ w272]
            frame False {
              # "Manipulator didnt request change"
            }
            frame True {
              # "Set height request to new value"
              n278 = case shown="0, Default" w272 {
                tunnel: [w274 w275 w276 w277 w278 w279] -> w273
                frame 0, Default {
                  n279 = global read "Lift Global.vi" "Cargo Zone 1 Height"() -> (w274:dbl)
                }
                frame 1 {
                  n280 = global read "Lift Global.vi" "Hatch Panel 1 Height"() -> (w275:dbl)
                }
                frame 2 {
                  n281 = global read "Lift Global.vi" "Cargo Zone 2 Height"() -> (w276:dbl)
                }
                frame 3 {
                  n282 = global read "Lift Global.vi" "Hatch Panel 2 Height"() -> (w277:dbl)
                }
                frame 4 {
                  n283 = global read "Lift Global.vi" "Cargo Zone 3 Height"() -> (w278:dbl)
                }
                frame 5 {
                  n284 = global read "Lift Global.vi" "Hatch Panel 3 Height"() -> (w279:dbl)
                }
              }
              n285 = global write "Lift Global.vi" "Requested Height"(w273) -> ()
            }
          }
          n286 = global write "Lift Global.vi" "Lift Auto Position"(w266) -> ()
          n287 = feedback-in #14(w266) -> ()
        }
        frame 0 {
          # "Manip pressing up on Dpad, or controller not plugged in"
          n288 = global read "Lift Global.vi" "Requested Height"() -> (w301:dbl)
          n289 = Add(x=w301, y=1.75) -> (x+y=w300:dbl)
          n290 = Greater?(x=w300, y=103.0) -> (0:w302:bool)
          n291 = Select(t=w301, s=w302, f=w300) -> (s? t:f=w303:dbl)
          n292 = global write "Lift Global.vi" "Requested Height"(w303) -> ()
        }
        frame 180 {
          # "Manip pressing down on Dpad"
          n293 = global read "Lift Global.vi" "Requested Height"() -> (w306:dbl)
          n294 = Add(x=w306, y=-1.0) -> (x+y=w308:dbl)
          n295 = Less?(x=w308, y=0.0) -> (x < y?=w309:bool)
          n296 = Select(t=w306, s=w309, f=w308) -> (s? t:f=w307:dbl)
          n297 = global write "Lift Global.vi" "Requested Height"(w307) -> ()
        }
        frame 90 {
          # "Go to Cargo in Cargo Ship Height"
          # "Right on D-Pad"
          n298 = global read "Lift Global.vi" "Cargo Ship Height"() -> (w312:dbl)
          n299 = global write "Lift Global.vi" "Requested Height"(w312) -> ()
        }
        frame 270 {
          # "Go to Hatch Level 1 Height"
          # "Left on D-Pad"
          n300 = global read "Lift Global.vi" "Hatch Panel 1 Height"() -> (w313:dbl)
          n301 = global write "Lift Global.vi" "Requested Height"(w313) -> ()
        }
        frame -100, Default {
        }
      }
    }
    frame Enabled {
    }
  }
  n302 = case shown="True" w1 {
    tunnel: w78 -> [w318 _]
    tunnel: [w317 w330] -> w77
    tunnel: [w316 w331] -> w76
    tunnel: w6 -> [w315 w328]
    tunnel: w5 -> [w314 w329]
    frame False {
      # "Non Visoin Track"
      n303 = case shown="True" w318 {
        tunnel: w314 -> [w320 w325]
        tunnel: [w320 w324] -> w317
        tunnel: [w319 w323] -> w316
        tunnel: w315 -> [w319 w322]
        frame False {
        }
        frame True {
          w321 = 0.65 ("Y Slower")
          n304 = Multiply(x=w322, y=w321) -> (x*y=w323:dbl)
          n305 = Multiply(x=w325, y=w321) -> (x*y=w324:dbl)
        }
      }
    }
    frame True {
      # "Vision Track"
      n306 = Multiply(x=w328, y=0.65 ("Y Slower")) -> (x*y=w331:dbl)
      n307 = Multiply(x=w329, y=0.7 ("Y Slower")) -> (x*y=w330:dbl)
    }
  }
  n308 = case shown="True" w64 {
    tunnel: w63 -> [w333 _]
    frame False {
      n309 = feedback #16() -> (w334:bool)  [unwired: 1 in]
      n310 = feedback-in #16(w333) -> ()
      n311 = Greater?(x=w333, y=w334) -> (0:w332:bool)
      n312 = case shown="True" w332 {
        frame False {
        }
        frame True {
          n313 = global read "Drive Train Global.vi" "Gyro Information"() -> (w341:T4)
          n314 = Unbundle By Name(w341) -> ("Yaw"=w338:dbl)
          n315 = Add(x=w338, y=180.0) -> (x+y=w337:dbl)
          n316 = Divide(x=w337, y=90.0) -> (x/y=w339:dbl)
          n317 = Round To Nearest(number=w339) -> (nearest integer value=w335:dbl)
          n318 = case shown="1" w335 {
            frame 0, Default {
              n319 = global write "Drive Train Global.vi" "Angle to Lock To"(180.0 ("Angle to Lock To")) -> ()
            }
            frame 1 {
              n320 = global write "Drive Train Global.vi" "Angle to Lock To"(270.0 ("Angle to Lock To")) -> ()
            }
            frame 2 {
              n321 = global write "Drive Train Global.vi" "Angle to Lock To"(0.0 ("Angle to Lock To")) -> ()
            }
            frame 3 {
              n322 = global write "Drive Train Global.vi" "Angle to Lock To"(90.0 ("Angle to Lock To")) -> ()
            }
            frame 4 {
              n323 = global write "Drive Train Global.vi" "Angle to Lock To"(180.0 ("Angle to Lock To")) -> ()
            }
          }
        }
      }
    }
    frame True {
      n324 = global read "Drive Train Global.vi" "Gyro Information"() -> (w355:T4)
      n325 = Unbundle By Name(w355) -> ("Cont Yaw"=w353:dbl)
      n326 = Quotient & Remainder(x=w353, y=360.0) -> (x-y*floor(x/y)=w351:dbl)  [unwired: 1 out]
      n327 = Divide(x=w351, y=60.0) -> (x/y=w347:dbl)
      n328 = In Range and Coerce(upper limit=1.5, x=w347, lower limit=0.0) -> (In Range?=w348:bool)  [unwired: 1 out]
      n329 = case shown="False" w348 {
        tunnel: w347 -> [w356 _]
        frame False {
          n330 = In Range and Coerce(upper limit=3.0, x=w356, lower limit=1.5) -> (In Range?=w357:bool)  [unwired: 1 out]
          n331 = case shown="True" w357 {
            tunnel: w356 -> [w362 _]
            tunnel: w356 -> [w360 _]
            frame False {
              n332 = In Range and Coerce(upper limit=4.5, x=w362, lower limit=3.0) -> (In Range?=w361:bool)  [unwired: 1 out]
              n333 = case shown="False" w361 {
                tunnel: w360 -> [w366 _]
                frame False {
                  n334 = In Range and Coerce(upper limit=6.0, x=w366, lower limit=4.5) -> (In Range?=w365:bool)  [unwired: 1 out]
                  n335 = case shown="True" w365 {
                    frame False {
                    }
                    frame True {
                      n336 = global write "Drive Train Global.vi" "Angle to Lock To"(330.0 ("Angle to Lock To")) -> ()
                    }
                  }
                }
                frame True {
                  n337 = global write "Drive Train Global.vi" "Angle to Lock To"(210.0 ("Angle to Lock To")) -> ()
                }
              }
            }
            frame True {
              n338 = global write "Drive Train Global.vi" "Angle to Lock To"(150.0 ("Angle to Lock To")) -> ()
            }
          }
        }
        frame True {
          n339 = global write "Drive Train Global.vi" "Angle to Lock To"(30.0 ("Angle to Lock To")) -> ()
        }
      }
    }
  }
  n340 = Subtract(x=w75, y=w67) -> (x-y=w74:dbl)
  n341 = Negate(x=w67) -> (-x=w68:dbl)
  n342 = Divide(x=w74, y=w68) -> (x/y=w72:dbl)
  n343 = Subtract(x=w73, y=w69) -> (x-y=w71:dbl)
  n344 = Multiply(x=w72, y=w71) -> (x*y=w70:dbl)
  n345 = Add(x=w70, y=w69) -> (x+y=w26:dbl)
  n346 = global read "Manipulator Controller Global.vi" "Options / Start"() -> (w50:bool)
  n347 = global read "Manipulator Controller Global.vi" "Share / Select"() -> (w51:bool)
  n348 = Multiply(x=w26, y=w13) -> (x*y=w84:dbl)
  n349 = Multiply(x=w26, y=w76) -> (x*y=w56:dbl)
  n350 = Multiply(x=w26, y=w77) -> (x*y=w49:dbl)
  n351 = Negate(x=w49) -> (-x=w48:dbl)
  n352 = global read "Driver Controller Global.vi" "Driver Right Bumper"() -> (w81:bool)
  n353 = global read "Driver Controller Global.vi" "Driver Left Bumper"() -> (w58:bool)
  n354 = global write "Drive Train Global.vi" "Y Command"(w48) -> ()
  n355 = Multiply(x=0.5, y=w84) -> (x*y=w83:dbl)
  n356 = Select(t=w83, s=w81, f=w84) -> (s? t:f=w57:dbl)
  n357 = global write "HAB Climber Global.vi" "HAB Retract"(w50) -> ()
  n358 = global write "HAB Climber Global.vi" "HAB Extend"(w51) -> ()
  n359 = case shown="False" w58 {
    tunnel: w56 -> [w374 w378]
    tunnel: [w374 w376] -> w55
    tunnel: w26 -> [_ w375]
    frame False {
      # "Driver not attepting to camera track, be normal"
      n360 = global write "Driver Controller Global.vi" "Output On"(FALSE ("Rumble Controller?")) -> ()
    }
    frame True {
      # "Driver wants to camera track"
      n361 = global read "Robot Global Data.vi" "Limelight Data"() -> (w380:T6)
      n362 = Unbundle By Name(w380) -> ("validTarget"=w379:dbl, "offsetAngle H"=w377:dbl)
      n363 = case shown="0, Default" w379 {
        tunnel: w378 -> [w383 _ _]
        tunnel: w377 -> [_ w388 w393]
        tunnel: [w383 w387 w394] -> w376
        tunnel: w375 -> [_ w385 _]
        frame 0, Default {
          # "No Valid Target, keep using driver controls\nand rumble controller so knows not tracking"
          n364 = global write "Driver Controller Global.vi" "Rumble Right"(1.0 ("Rumble Amount")) -> ()
          n365 = global write "Driver Controller Global.vi" "Rumble Left"(1.0 ("Rumble Amount")) -> ()
          n366 = global write "Driver Controller Global.vi" "Output On"(TRUE ("Rumble Controller?")) -> ()
        }
        frame 1 {
          # "There is a valid target, track target"
          n367 = call-poly <vilib>:"PID.vi"("output range"=cluster{"output high":dbl, "output low":dbl} {"output high"=1.0, "output low"=-1.0}, "PID gains"="Camera Tracking", "setpoint"=w388) -> ("output"=w386:dbl)  [unwired: 7 in, 1 out]
          n368 = global write "Driver Controller Global.vi" "Output On"(FALSE ("Rumble Controller?")) -> ()
          n369 = Multiply(x=w385, y=w386) -> (x*y=w387:dbl)
        }
        frame 2 {
          n370 = Multiply(x=0.1, y=w393) -> (x*y=w394:dbl)
        }
      }
    }
  }
  n371 = global write "Drive Train Global.vi" "Z Command"(w57) -> ()
  n372 = global write "Drive Train Global.vi" "X Command"(w55) -> ()
